vi "Tusk.UnwrapQueueMessage.vi"(7 "timeout in ms (-1)":i32=-1, 8 "error in (no error)":errorcluster, 11 "Tusk in":refnum<class "Tusk.lvclass">) -> (0 "error out":errorcluster, 1 "Data":variant, 2 "Message":string, 3 "Tusk out":refnum<class "Tusk.lvclass">, 4 "Sender":string, 5 "Time Sent":timestamp)   [LabVIEW 2018, in "Application.lvlib" / "Tusk.lvclass"]
uses:
  Tusk.lvclass
  Tusk.lvclass/Tusk.ctl
  Message Class/Message.lvclass/Message.ctl
  Message Class/VIs/Unwrap Message.vi
  Keywords Class/VIs/{Self}.vi
  <vilib>/Utility/error.llb/Trim Whitespace.vi
  Message Class/Message.lvclass
  Keywords Class/Keywords.lvclass
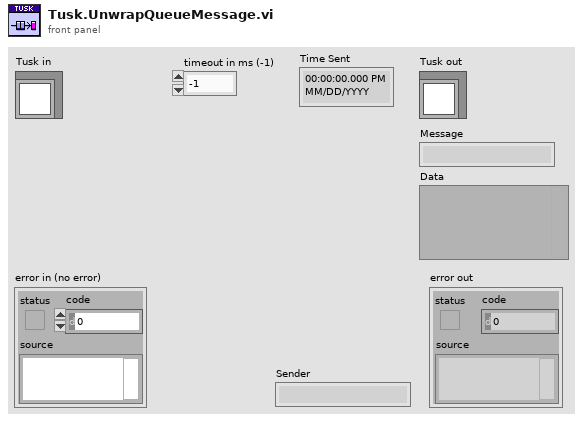
[diagram p1: front panel]
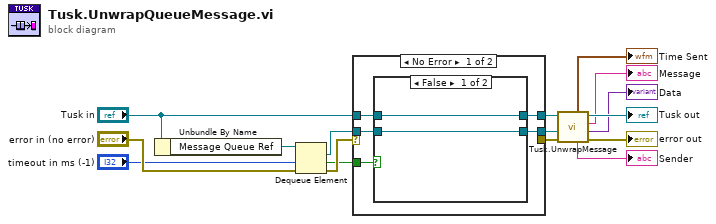
[diagram p0: block diagram]
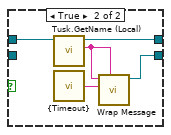
[diagram p2: hidden frame]
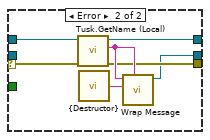
[diagram p3: hidden frame]
diagram:
  n1 = Unbundle By Name("Tusk in") -> ("Message Queue Ref"=w14:refnum<queue>)
  n2 = Dequeue Element(queue=w14, timeout in ms (-1)="timeout in ms (-1)", error in (no error)="error in (no error)") -> (element=w4:refnum<class "Message.lvclass">, timed out?=w7:bool, error out=w16:errorcluster)  [unwired: 1 out]
  n3 = case shown="No Error" w16 {
    selector: w16 -> [_ w32]
    tunnel: w7 -> [w21 _]
    tunnel: "Tusk in" -> [w20 w34]
    tunnel: [w19 w33] -> w5
    tunnel: [w18 w29] -> w1
    tunnel: w4 -> [w17 _]
    tunnel: [_ w31] -> w2
    frame No Error {
      n4 = case shown="False" w21 {
        tunnel: w20 -> [w23 w28]
        tunnel: [w23 w27] -> w19
        tunnel: [w22 w25] -> w18
        tunnel: w17 -> [w22 _]
        frame False {
        }
        frame True {
          n5 = call "Tusk.GetName (Local).vi"("Tusk in"=w28) -> ("Name(Local)"=w26:string, "Tusk out"=w27:refnum<class "Tusk.lvclass">)  [unwired: 8 in, 1 out]
          n6 = call "{Timeout}.vi"() -> ("Word"=w24:string)  [unwired: 6 in]
          n7 = call "Wrap Message.vi"("Sender"=w26, "Message"=w24, "Recipient"=w26) -> ("Message out"=w25:refnum<class "Message.lvclass">)  [unwired: 7 in, 1 out]
        }
      }
    }
    frame Error {
      n8 = call "Tusk.GetName (Local).vi"("error in (no error)"=w32, "Tusk in"=w34) -> ("error out"=w31:errorcluster, "Name(Local)"=w35:string, "Tusk out"=w33:refnum<class "Tusk.lvclass">)  [unwired: 7 in]
      n9 = call "{Destructor}.vi"() -> ("Word"=w30:string)  [unwired: 6 in]
      n10 = call "Wrap Message.vi"("Sender"=w35, "Message"=w30, "Recipient"=w35) -> ("Message out"=w29:refnum<class "Message.lvclass">)  [unwired: 7 in, 1 out]
    }
  }
  n11 = call "Tusk.UnwrapMessage.vi"("error in (no error)"=w2, "Message"=w1, "Tusk in"=w5) -> ("error out"=→"error out":errorcluster, "Data"=→"Data":variant, "Message"=→"Message":string, "Tusk out"=→"Tusk out":refnum<class "Tusk.lvclass">, "Sender"=→"Sender":string, "Time Sent"=→"Time Sent":timestamp)  [unwired: 3 in]
